vi "measure(SubVI).vi"(0 "config in":T1={"initialize"=enum."SR830", "6221"={"6221 Resource"="GPIB0::24::INSTR", "Delta status"=FALSE, "电流"=0.0}, "SR830+6221"={"source"=0, "阻抗"=0.0, "量程入 4"=0, "量程入 3"=0, "量程入 2"=0, "量程入 1"=0, "SR830 2"=FALSE, "SR830 3"=FALSE, "SR830 4"=FALSE, "SR830 1"=FALSE, "VISA 1"="", "VISA 2"="", "VISA 3"="", "VISA 4"="", "Reserve 1"=0, "Reserve 2"=-1, "Reserve 3"=-1, "Reserve 4"=-1, "量程"=enum."量程每次测量会判定"}, "2400"={"2400"=FALSE, "VISA"=""}, "ch"={"ch"=[], "current"=[], "change?"=[], "holding current\nwhen change ch?"=FALSE}, "Instrument"={"335 Resource"="GPIB0::24::INSTR", "Input (0:A)"=0, "Instrument Type"=enum."SVSM", "quantum design"=refnum, "Heater Output (1:1)"=1, "semaphore"=refnum, "TCP master instance"=refnum, "335 Status"=refnum, "M24C Resource"="GPIB0::24::INSTR", "4G supply"="GPIB0::24::INSTR", "Temp Status 24C"=refnum, "Temp"=refnum, "9T信号"=refnum, "4g supply status"=refnum}, "Aborting"=refnum, "数据文件"=refnum} {"Instrument"."Input (0:A)" items=["A", "B"]; "Instrument"."Heater Output (1:1)" items=["1"=1, "2"=2]; "SR830+6221"."Reserve 4" items=["Auto Reserve"=-1, "High Reserve"=0, "Normal"=1, "Low Noise"=2]; "SR830+6221"."Reserve 3" items=["Auto Reserve"=-1, "High Reserve"=0, "Normal"=1, "Low Noise"=2]; "SR830+6221"."Reserve 2" items=["Auto Reserve"=-1, "High Reserve"=0, "Normal"=1, "Low Noise"=2]; "SR830+6221"."Reserve 1" items=["量程每次测量会判定", "量程不变为设定值"]; "SR830+6221"."source" items=["SR830 1", "SR830 2", "SR830 3", "SR830 4"]}, 5 "ch":i32, 7 "current":dbl, 9 "change?":bool, 11 "error in (no error)":errorcluster) -> (4 "data":string[](array[string]), 6 "config out":T1={"initialize"=enum."SR830", "6221"={"6221 Resource"="GPIB0::24::INSTR", "Delta status"=FALSE, "电流"=0.0}, "SR830+6221"={"source"=0, "阻抗"=0.0, "量程入 4"=0, "量程入 3"=0, "量程入 2"=0, "量程入 1"=0, "SR830 2"=FALSE, "SR830 3"=FALSE, "SR830 4"=FALSE, "SR830 1"=FALSE, "VISA 1"="", "VISA 2"="", "VISA 3"="", "VISA 4"="", "Reserve 1"=0, "Reserve 2"=-1, "Reserve 3"=-1, "Reserve 4"=-1, "量程"=enum."量程每次测量会判定"}, "2400"={"2400"=FALSE, "VISA"=""}, "ch"={"ch"=[], "current"=[], "change?"=[], "holding current\nwhen change ch?"=FALSE}, "Instrument"={"335 Resource"="GPIB0::24::INSTR", "Input (0:A)"=0, "Instrument Type"=enum."SVSM", "quantum design"=refnum, "Heater Output (1:1)"=1, "semaphore"=refnum, "TCP master instance"=refnum, "335 Status"=refnum, "M24C Resource"="GPIB0::24::INSTR", "4G supply"="GPIB0::24::INSTR", "Temp Status 24C"=refnum, "Temp"=refnum, "9T信号"=refnum, "4g supply status"=refnum}, "Aborting"=refnum, "数据文件"=refnum} {"Instrument"."Input (0:A)" items=["A", "B"]; "Instrument"."Heater Output (1:1)" items=["1"=1, "2"=2]; "SR830+6221"."Reserve 4" items=["Auto Reserve"=-1, "High Reserve"=0, "Normal"=1, "Low Noise"=2]; "SR830+6221"."Reserve 3" items=["Auto Reserve"=-1, "High Reserve"=0, "Normal"=1, "Low Noise"=2]; "SR830+6221"."Reserve 2" items=["Auto Reserve"=-1, "High Reserve"=0, "Normal"=1, "Low Noise"=2]; "SR830+6221"."Reserve 1" items=["量程每次测量会判定", "量程不变为设定值"]; "SR830+6221"."source" items=["SR830 1", "SR830 2", "SR830 3", "SR830 4"]}, 15 "error out":errorcluster)   [LabVIEW 2019, in "SubVI.lvlib"]
uses:
  SubVI.lvlib
  config.ctl
  <vilib>/NI/Modbus Library/API/Master/Modbus Master.lvclass
  initialize.ctl
  Instrument.ctl
  Instrument Type.ctl
  lib/QDInstrument.dll
  335 state.ctl
  9T mag field stauts.ctl
  lib/Keithley 24XX/Public/Data/Read (Single Point).vi
  lib/Keithley 24XX/Keithley 24XX.lvlib
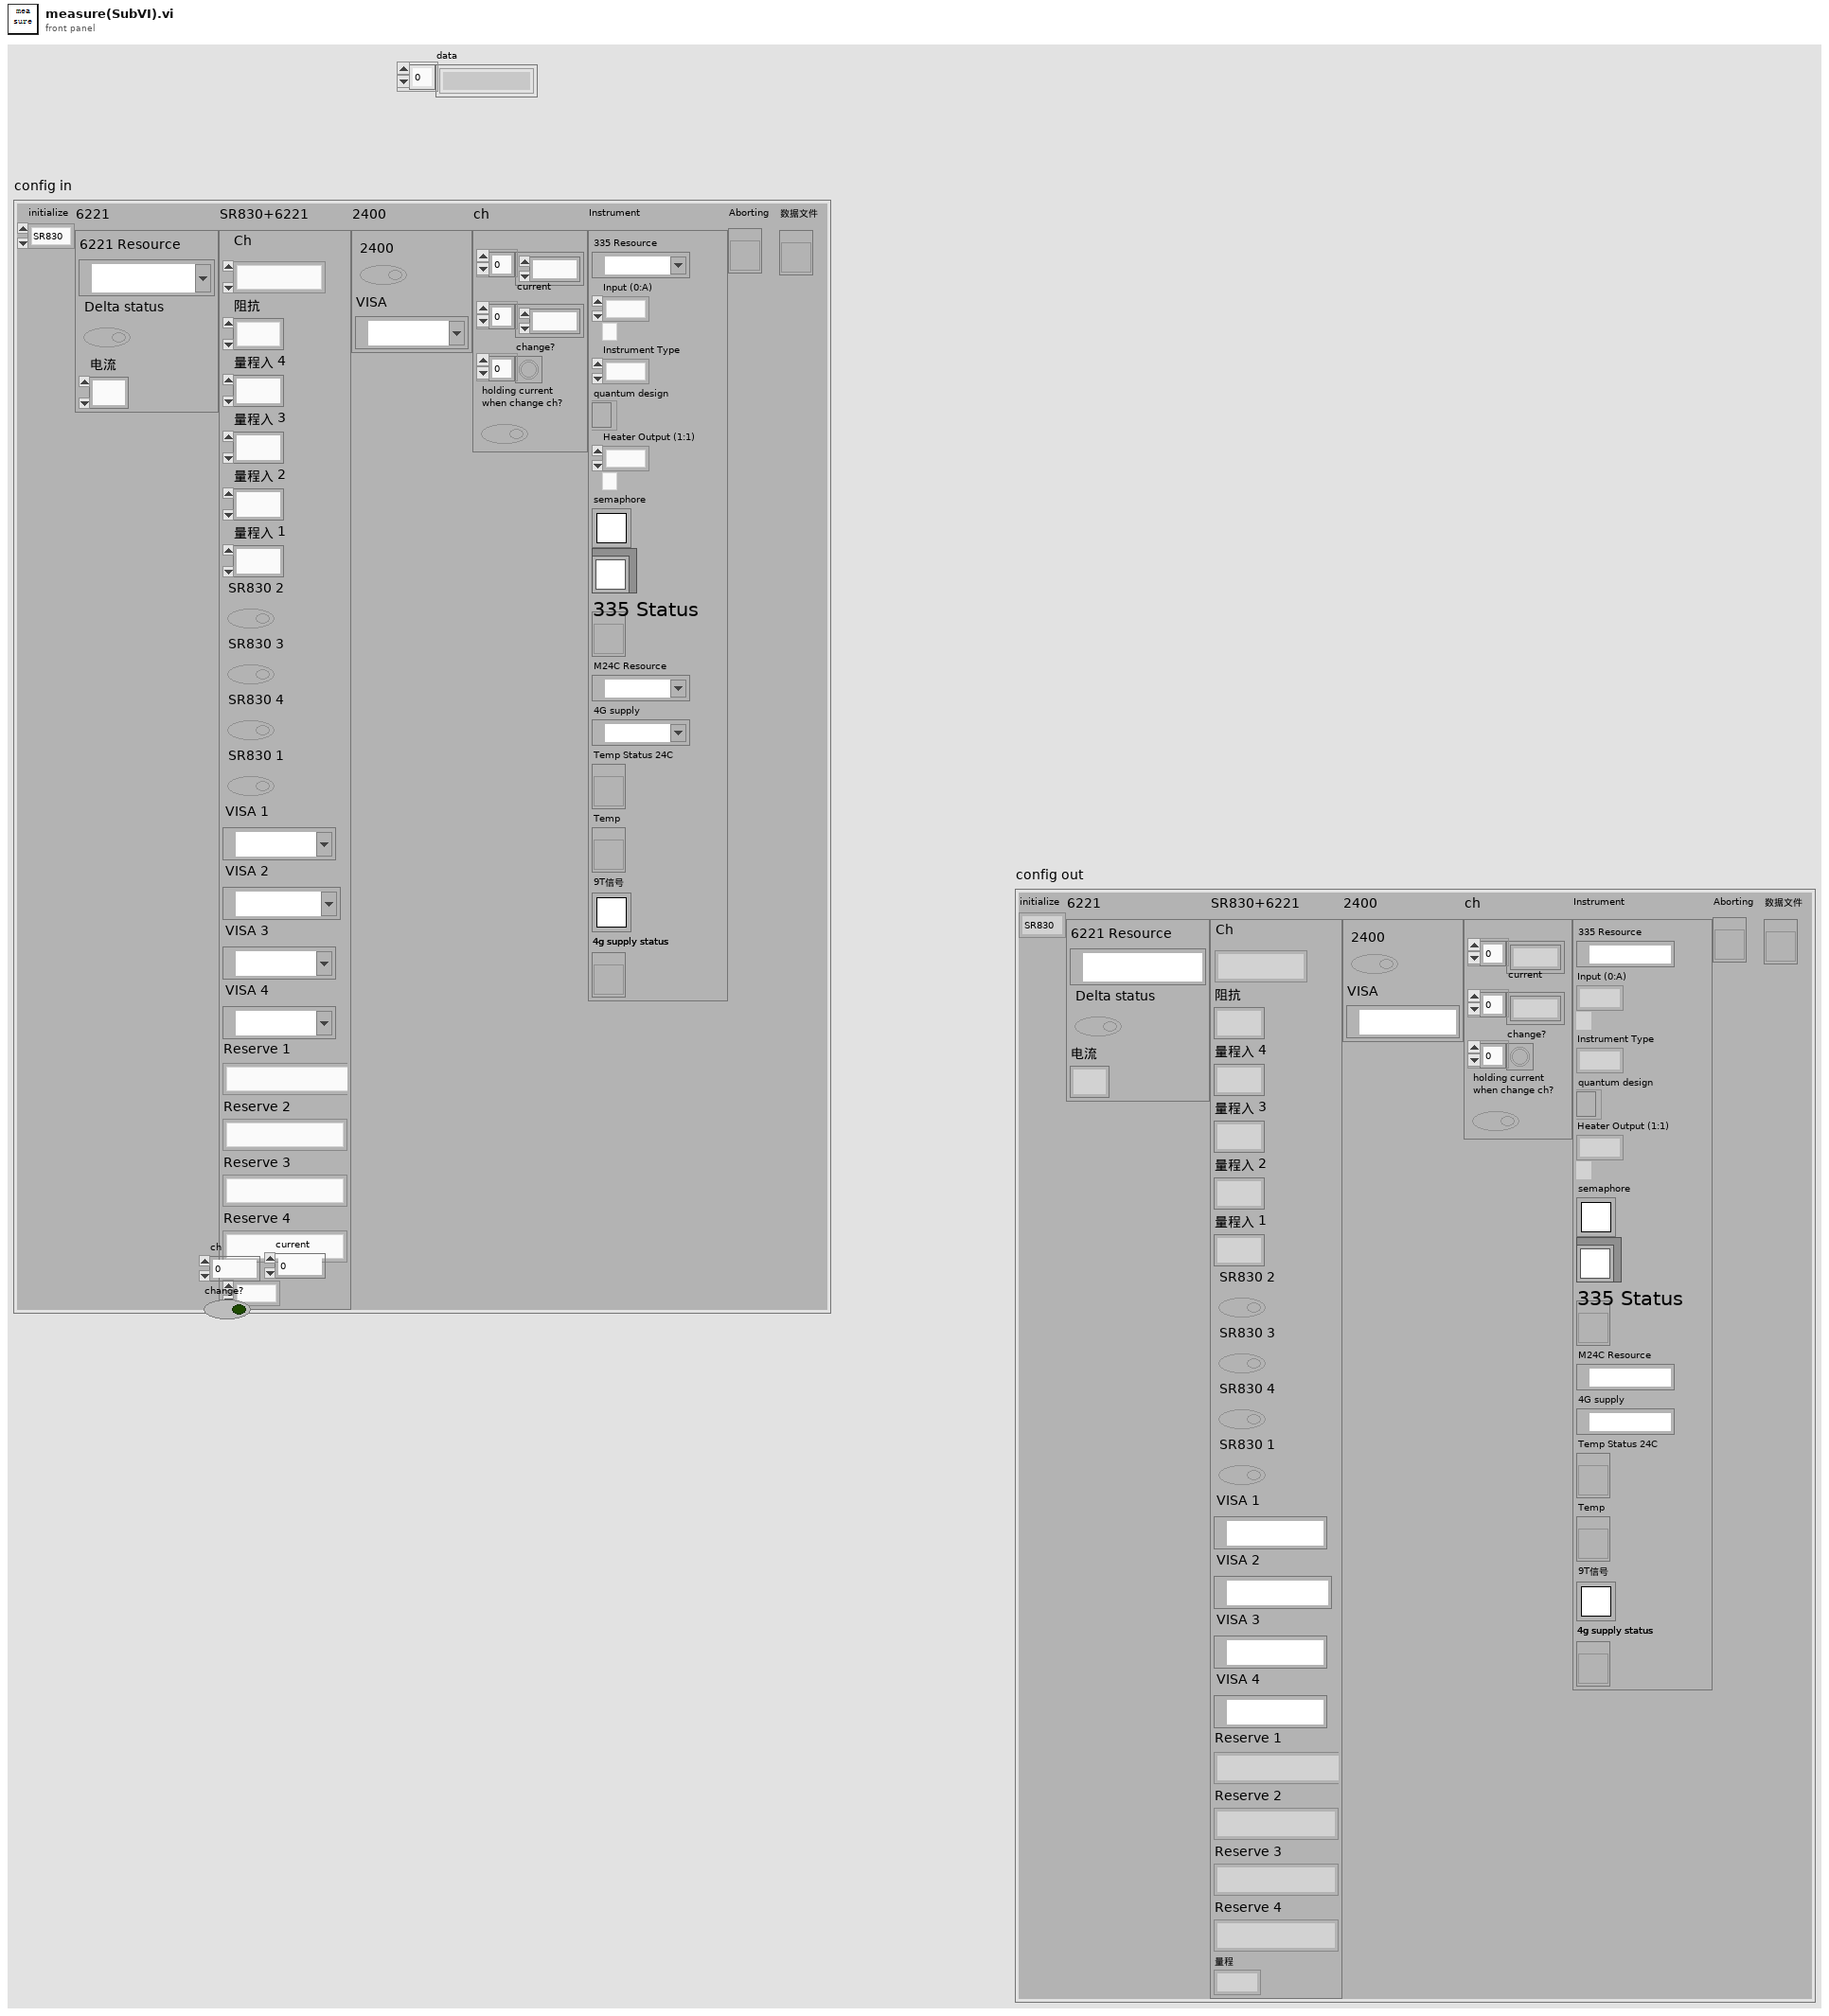
[diagram p1: front panel]
types:
  T1 = typedef "config.ctl" = cluster{"initialize":T2, "6221":cluster{"6221 Resource":refnum<visa-resource-name>, "Delta status":bool, "电流":dbl}, "SR830+6221":cluster{"source":u16, "阻抗":dbl, "量程入 4":i32, "量程入 3":i32, "量程入 2":i32, "量程入 1":i32, "SR830 2":bool, "SR830 3":bool, "SR830 4":bool, "SR830 1":bool, "VISA 1":refnum<visa-resource-name>, "VISA 2":refnum<visa-resource-name>, "VISA 3":refnum<visa-resource-name>, "VISA 4":refnum<visa-resource-name>, "Reserve 1":i16, "Reserve 2":i16, "Reserve 3":i16, "Reserve 4":i16, "量程":enum16{"量程每次测量会判定", "量程不变为设定值"}}, "2400":cluster{"2400":bool, "VISA":refnum<visa-resource-name>}, "ch":cluster{"ch":i32[], "current":dbl[], "change?":bool[], "holding current\nwhen change ch?":bool}, "Instrument":T3, "Aborting":refnum<vi>, "数据文件":refnum<vi>}
  T2 = typedef "initialize.ctl" = enum16{"SR830", "keithley6221-SR830", "Delta", "Delta-tunnelling", "keithley6221-2182-DC"}
  T3 = typedef "Instrument.ctl" = cluster{"335 Resource":refnum<visa-resource-name>, "Input (0:A)":u16, "Instrument Type":T4, "quantum design":refnum<k24>, "Heater Output (1:1)":u16, "semaphore":T5, "TCP master instance":refnum<class "Modbus Master.lvclass">, "335 Status":refnum<vi>, "M24C Resource":refnum<visa-resource-name>, "4G supply":refnum<visa-resource-name>, "Temp Status 24C":refnum<vi>, "Temp":refnum<vi>, "9T信号":T5, "4g supply status":refnum<vi>}
  T4 = typedef "Instrument Type.ctl" = enum16{"PPMS", "VersaLab", "DynaCool", "SVSM", "PPMS-Rotate", "Lakeshore335", "9T mag"}
  T5 = typedef "Semaphore RefNum" = refnum<k1>
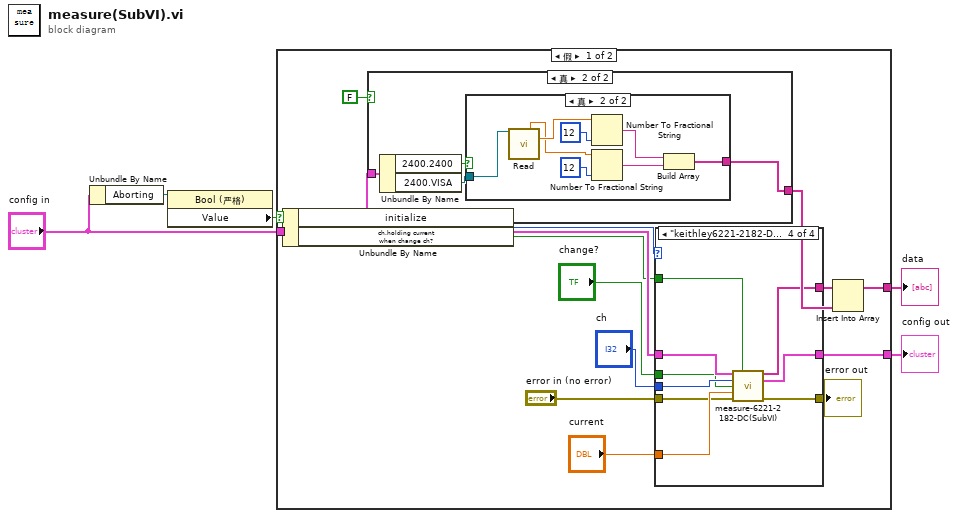
[diagram p0: block diagram]
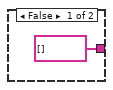
[diagram p2: hidden frame]
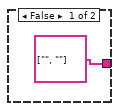
[diagram p3: hidden frame]
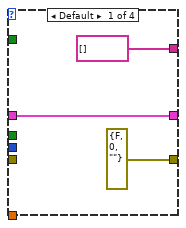
[diagram p4: hidden frame]
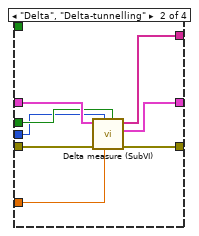
[diagram p5: hidden frame]
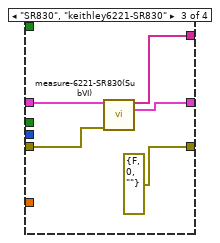
[diagram p6: hidden frame]
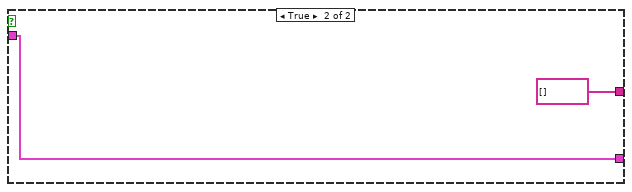
[diagram p7: hidden frame]
diagram:
  n1 = Unbundle By Name("config in") -> ("Aborting"=w4:refnum<vi>)
  n2 = property class="Bool (严格)"(reference=w4) -> ("Value"=w3:bool)  [unwired: 1 in, 2 out]
  n3 = case shown="假" w3 {
    tunnel: "config in" -> [w12 w59]
    tunnel: [w11 w59] -> w2
    tunnel: [w10 string[] [] ("输出数组")] -> w1
    frame False {
      n4 = Unbundle By Name(w12) -> ("initialize"=w13:T2, "ch.holding current\nwhen change ch?"=w6:bool)
      n5 = case shown="真" FALSE {
        tunnel: [string[] [] w21] -> w15
        tunnel: w12 -> [_ w20]
        frame False {
        }
        frame True {
          n6 = Unbundle By Name(w20) -> ("2400.2400"=w23:bool, "2400.VISA"=w22:refnum<visa-resource-name>)
          n7 = case shown="真" w23 {
            tunnel: w22 -> [_ w32]
            tunnel: [string[] ["", ""] w25] -> w21
            frame False {
            }
            frame True {
              n8 = call-poly "Read.vi"("VISA resource name"=w32) -> ("Voltage"=w29:sgl, "Current"=w30:sgl)  [unwired: 8 in, 5 out]
              n9 = Number To Fractional String(number=w30, precision (6)=i16 12 ("精度(6)")) -> (F-format string=w27:string)  [unwired: 2 in]
              n10 = Number To Fractional String(number=w29, precision (6)=i16 12 ("精度(6)")) -> (F-format string=w26:string)  [unwired: 2 in]
              n11 = Build Array(w27, w26) -> (w25:string[])
            }
          }
        }
      }
      n12 = case shown="\"keithley6221-2182-DC\"" w13 {
        tunnel: [string[] [] w43 w46 w56] -> w16
        tunnel: "error in (no error)" -> [_ w42 w48 w50]
        tunnel: [errorcluster {"status"=FALSE, "code"=0, "source"=""} ("error out") w41 errorcluster {"status"=FALSE, "code"=0, "source"=""} ("error out") w54] -> w17
        tunnel: w12 -> [w33 w40 w45 w57]
        tunnel: [w33 w39 w44 w55] -> w11
        tunnel: "change?" -> [_ w38 _ w51]
        tunnel: "ch" -> [_ w37 _ w53]
        tunnel: "current" -> [_ w36 _ w52]
        tunnel: w6 -> [_ _ _ w49]
        frame Default {
        }
        frame "Delta", "Delta-tunnelling" {
          n13 = call "Delta measure (SubVI).vi"("change?"=w38, "current"=w36, "ch"=w37, "错误输入（无错误）"=w42, "输出簇 2"=w40) -> ("错误输出"=w41:errorcluster, "输出簇 3"=w39:T1, "数组"=w43:string[])  [unwired: 4 in]
        }
        frame "SR830", "keithley6221-SR830" {
          n14 = call "measure-6221-SR830(SubVI).vi"("输入簇"=w45, "错误输入"=w48) -> ("输出数组"=w46:string[], "输出簇"=w44:T1)  [unwired: 11 in, 1 out]
        }
        frame "keithley6221-2182-DC" {
          n15 = call "measure-6221-2182-DC(SubVI).vi"("输入簇"=w57, "Holding current？"=w49, "ch"=w53, "change?"=w51, "current"=w52, "错误输入"=w50) -> ("输出数组"=w56:string[], "输出簇"=w55:T1, "错误输出"=w54:errorcluster)  [unwired: 7 in]
        }
      }
      "error out" <- w17
      n16 = Insert Into Array(array=w16, new element=w15) -> (w10:string[])  [unwired: 1 in]
    }
    frame True {
    }
  }
  "config out" <- w2
  "data" <- w1
